vi "Command Editor Dialog _202503.vi"(7 "Name (\"\" to Use Uuid)":string="Event CSM Tiny", 8 "Error In":errorcluster caption="Error in (no error)", 11 "Command":string="UI: Front Panel State >> Open -@ abc") -> (0 "Error Out":errorcluster, 3 "Command Out":string)   [LabVIEW 2017]
uses:
  user.lib/_NEVSTOP/Communicable State Machine(CSM)/AdvanceAPI/CSM - Keywords.vi
  user.lib/_NEVSTOP/Communicable State Machine(CSM)/AdvanceAPI/CSM - Break Down Multiple States String.vi
  user.lib/_NEVSTOP/Communicable State Machine(CSM)/AdvanceAPI/CSM - Compact Multiple States.vi
  user.lib/_NEVSTOP/Communicable State Machine(CSM)/_Polymophic/CSM - Replace Marks in Messages.vi
  user.lib/_NEVSTOP/Communicable State Machine(CSM)/_Polymophic/Add State(s) to Queue By BOOL(Element).vi
  user.lib/_NEVSTOP/Communicable State Machine(CSM)/_Polymophic/Build Message with Arguments(Auto Check).vi
  user.lib/_NEVSTOP/Communicable State Machine(CSM)/Communicable State Machine.lvlib
  user.lib/_NEVSTOP/Communicable State Machine(CSM)/_csmHelper/API with lvcsm Support/CSM-Helper API with lvcsm Support.lvlib
  user.lib/_NEVSTOP/Communicable State Machine(CSM)/_csmHelper/CSM-Helper.lvclass
  user.lib/_NEVSTOP/Communicable State Machine(CSM)/_Shared/CSM Shared.lvlib
panel:
  in  "UserDef State Only":bool
  in  "State":string(combo)
  in  "Argument":string(combo)
  in  "symbol":string(combo)
  in  "Target":string(combo)
  in  "Comments":string
  in  "CSM-VI":string(combo)
  out "current time":timestamp
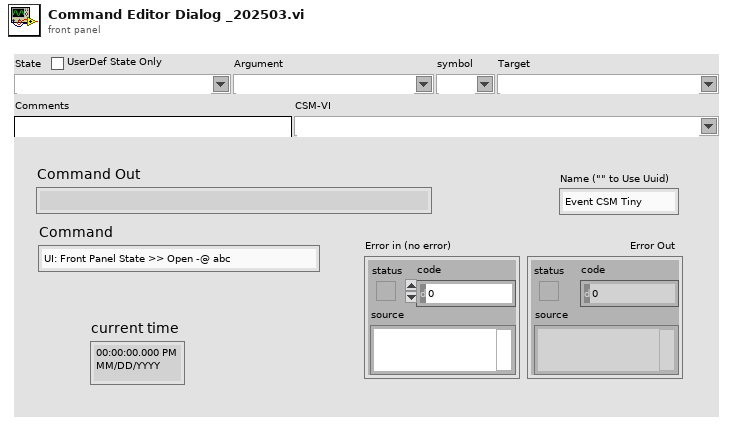
[diagram p1: front panel]
types:
  T1 = enum32{"Invalid", "Standard", "Closed", "Hidden", "Minimized", "Maximized"}
  T2 = enum32{"invalid app kind", "Development System", "Run Time System", "Student Edition", "Embedded LabVIEW", "Evaluation", "Custom"}
  T3 = enum8{"Enabled", "Disabled", "Disabled and Grayed Out"}
  T4 = typedef "Communicable State Machine.lvlib/_CSM_Response Source Message.ctl" = cluster{"‘State":string, "’Arguments":string, "’Error":errorcluster}
  T5 = typedef "eventvkey.ctl" = enum16{"ASCII", "Enter", "Return", "Shift", "Ctrl", "Alt", "Cmd", "Opt", "Caps", "NumLock", "Clear", "Break", "Up", "Down", "Left", "Right", "Insert", "Delete", "Home", "End", "PageUp", "PageDown", "Escape", "Help", "Pause", "ScrollLock", "F1", "F2", "F3", "F4", "F5", "F6", "F7", "F8", "F9", "F10", "F11", "F12", "F13", "F14", "F15", "F16", "F17", "F18", "F19", "F20", "F21", "F22", "F23", "F24", "Play", "VolumeUp", "VolumeDown", "Mute", "Two Byte Char"}
  T6 = cluster{"Shift":bool, "Ctrl":bool, "Alt":bool, "Cmd":bool, "Opt":bool}
  T7 = cluster{"Current VI Reference":refnum<vi>, "Close Panel on Exit?":bool}
  T8 = cluster{"Core":cluster{"Current VI Reference":refnum<vi>, "Close Panel on Exit?":bool}, "Command":string}
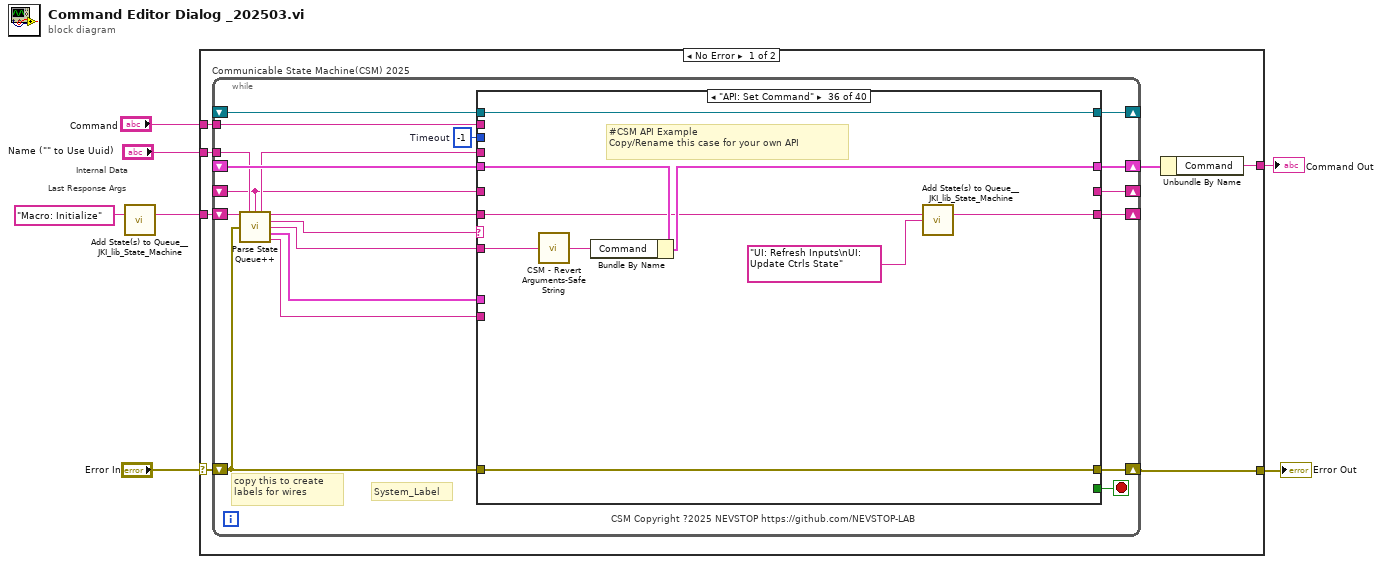
[diagram p0: block diagram]
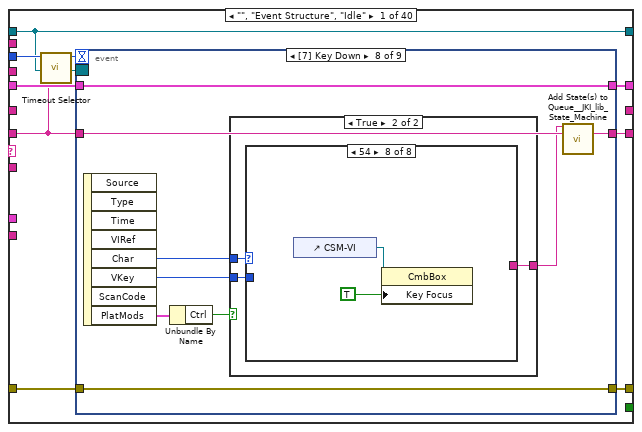
[diagram p2: hidden frame]
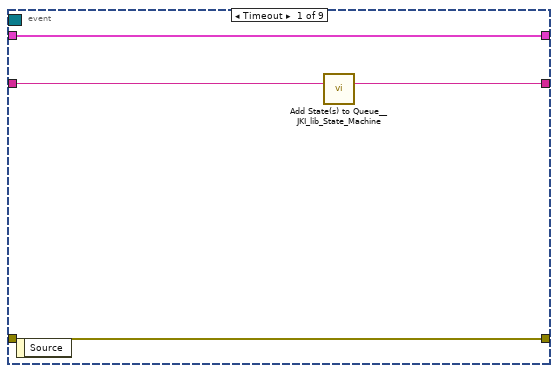
[diagram p3: hidden frame]
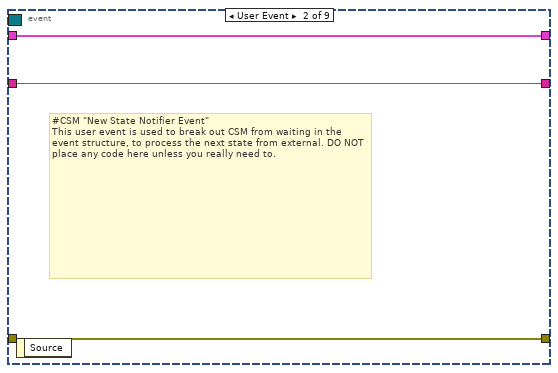
[diagram p4: hidden frame]
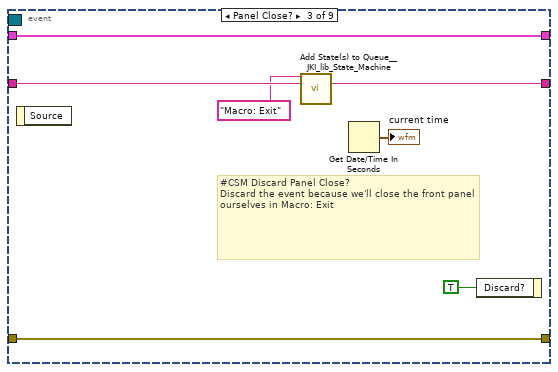
[diagram p5: hidden frame]
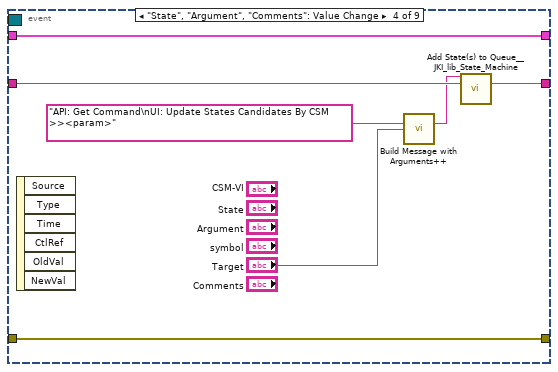
[diagram p6: hidden frame]
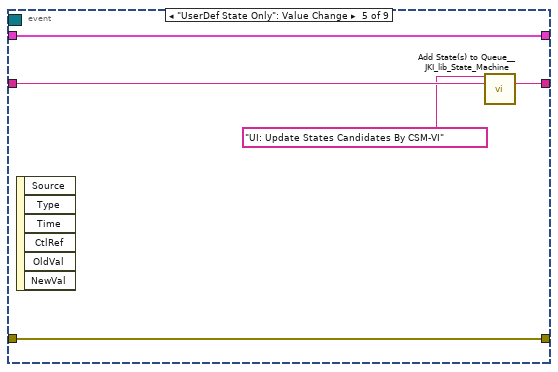
[diagram p7: hidden frame]
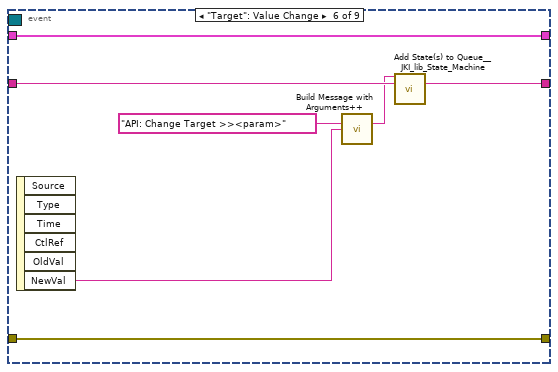
[diagram p8: hidden frame]
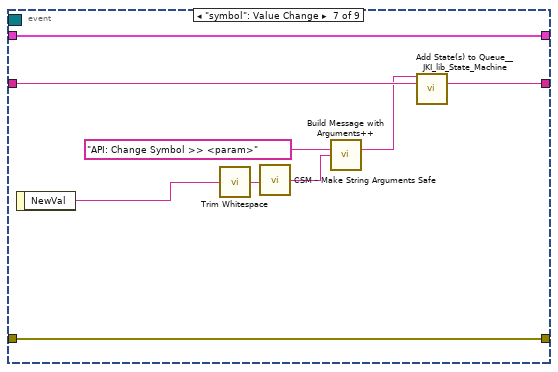
[diagram p9: hidden frame]
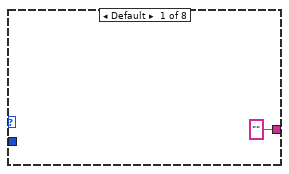
[diagram p11: hidden frame]
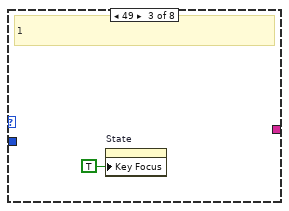
[diagram p13: hidden frame]
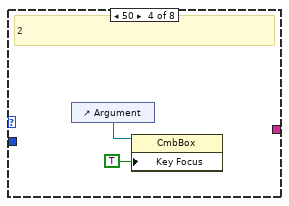
[diagram p14: hidden frame]
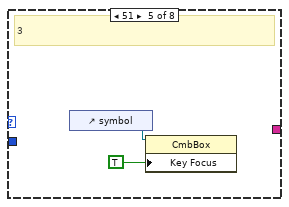
[diagram p15: hidden frame]
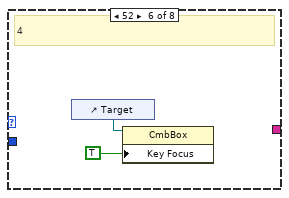
[diagram p16: hidden frame]
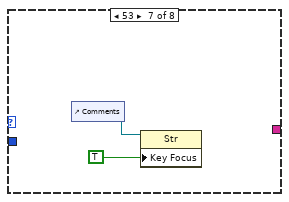
[diagram p17: hidden frame]
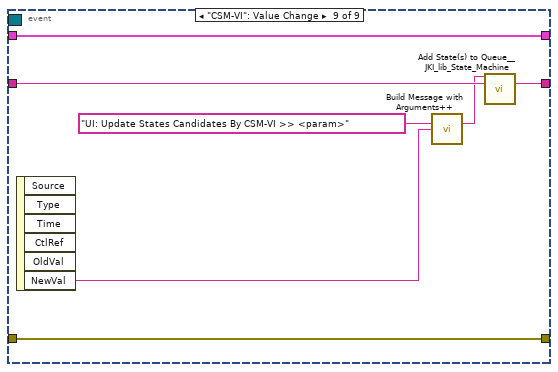
[diagram p18: hidden frame]
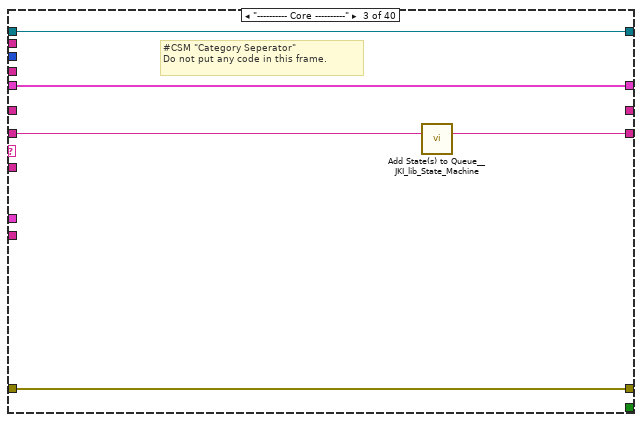
[diagram p20: hidden frame]
diagram:
  # "Last Response Args"
  # "Internal Data"
  n1 = call <vilib>:"Add State(s) to Queue__JKI_lib_State_Machine.vi"("State(s) in (\"\")"="Macro: Initialize" ("Init State(\"Macro: Initialize\")")) -> ("States Out"=w7:string)  [unwired: 14 in]
  n2 = case shown="No Error" "Error In" {
    selector: "Error In" -> [w11 w534]
    tunnel: w7 -> [w14 _]
    tunnel: "Name (\"\" to Use Uuid)" -> [w13 _]
    tunnel: [w12 w534] -> w4
    tunnel: [w9 w533] -> w1
    tunnel: "Command" -> [w8 w533]
    frame No Error {
      n3 = while "Communicable State Machine(CSM) 2025" {
        shift-right: [w29] -> w10
        shift-left: _ -> [w28]
        shift-right: [w32] -> w12
        shift-left: w11 -> [w26]
        shift-right: [w31] -> _
        shift-left: w14 -> [w33]
        tunnel: w13 -> [w22]
        shift-right: [w25] -> _
        shift-left: _ -> [w16]
        shift-right: [w24] -> _
        shift-left: _ -> [w23]
        tunnel: w8 -> [w15]
        stop <- w30 stop-if-true
        w27 = -1  # Timeout
        # "copy this to create labels for wires"
        # "System_Label"
        # "CSM Copyright ?2025 NEVSTOP https://github.com/NEVSTOP-LAB"
        n4 = call "Parse State Queue++.vi"("State Queue"=w33, "Name (\"\" to Use UUID)"=w22, "Response Arguments"=w16, "Previous Error"=w26) -> ("Name Used"=w17:string, "Remaining States"=w34:string, "Current State"=w21:string, "Arguments"=w20:string, "Additional Information"=w19:T4, "Source CSM"=w18:string)  [unwired: 6 in]
        n5 = case shown="\"API: Set Command\"" w21 {
          selector: w21 -> [_ _ _ w128 _ _ _ _ _ _ _ _ _ _ _ _ _ _ _ _ _ _ _ _ _ _ _ _ _ _ _ _ _ _ _ _ _ _ _ _]
          tunnel: w34 -> [w35 w119 w125 w133 w140 w146 w169 w175 w182 w191 w204 w219 w225 w230 w237 w244 w249 w256 w260 w266 w272 w278 w298 w314 w383 w388 w395 w413 w422 w429 w445 w456 w462 w474 w477 w480 w501 w513 w523 w532]
          tunnel: w20 -> [_ _ _ _ _ w145 w164 w174 w181 w190 _ _ _ _ _ _ _ _ _ _ _ _ w293 w308 _ _ w397 w410 w419 w426 _ _ _ _ _ w482 _ w514 w520 _]
          tunnel: w28 -> [w42 w118 w122 w131 w139 w150 w170 w177 w184 w193 w203 w212 w223 w227 _ w239 w246 w255 w259 w263 w268 w281 w296 w310 w382 w387 w399 w412 w421 w428 w444 w453 w459 w471 w476 w486 w500 w516 w525 w529]
          tunnel: [w41 w120 w123 w126 w141 errorcluster {"status"=FALSE, "code"=0, "source"=""} ("error out") w165 w172 w179 w196 w205 w216 w222 w228 w234 w240 w247 w250 w258 w264 w270 w291 w294 w311 w384 w389 w400 w414 w423 w430 w446 w454 w460 w472 w478 w487 w502 w517 w526 w530] -> w32
          tunnel: w26 -> [w40 w120 w123 w134 w141 w147 w171 w173 w180 _ w205 w216 w222 w228 w234 w241 w247 _ w261 w264 w270 w291 w295 w312 w384 w389 w400 w414 w423 w430 w446 w454 w460 w472 w478 w487 w502 w517 w526 w530]
          tunnel: [w43 w119 w124 w132 w140 w142 w168 w178 w185 w192 w204 w218 w224 w229 w236 w243 w248 w256 w260 w265 w271 w279 w297 w313 w383 w388 w396 w413 w422 w429 w445 w455 w461 w473 w477 w481 w501 w512 w527 w531] -> w31
          tunnel: [_ _ _ _ _ _ TRUE _ _ _ _ _ TRUE _ _ _ _ _ _ _ _ _ _ _ _ _ _ _ _ _ _ _ _ _ _ _ _ _ _ _] -> w30
          tunnel: [w39 w118 w122 w131 w139 w150 w170 w177 w184 w194 w203 w217 w223 w227 w235 w239 w246 w255 w259 w263 w268 w281 w296 w310 w382 w387 w399 w412 w421 w428 w444 w453 w459 w471 w476 w484 w490 w516 w525 w529] -> w29
          tunnel: w27 -> [w38 _ _ _ _ _ _ _ _ _ _ _ _ _ _ _ _ _ _ _ _ _ _ _ _ _ _ _ _ _ _ _ _ _ _ _ _ _ _ _]
          tunnel: w18 -> [_ _ _ _ _ _ _ _ _ w188 _ _ _ _ _ _ _ _ _ _ _ _ _ _ _ _ _ _ _ _ _ _ _ _ _ _ _ _ _ _]
          tunnel: w19 -> [_ _ _ _ _ _ _ _ _ w195 _ _ _ _ _ _ _ _ _ _ _ _ _ _ _ _ _ _ _ _ _ _ _ _ _ _ _ _ _ _]
          tunnel: [_ _ _ "" w135 _ _ _ _ _ _ _ _ _ _ _ _ _ _ _ _ _ _ _ _ _ _ _ _ _ _ _ _ _ _ _ w495 _ _ _] -> w25
          tunnel: [w37 w117 w121 w129 w138 w149 w166 w176 w183 w197 w202 w206 w220 w226 w232 w238 w245 w254 w257 w262 w269 w290 w292 w307 w381 w386 w398 w411 w420 w427 w443 w452 w457 w464 w475 w485 w499 w515 w524 w528] -> w24
          tunnel: w23 -> [w37 w117 w121 w129 w138 w149 w166 w176 w183 w197 w202 w206 w220 w226 w232 w238 w245 _ w257 w262 w269 w290 w292 w307 w381 w386 w398 w411 w420 w427 w443 w452 w457 w464 w475 w485 w499 w515 w524 w528]
          tunnel: w17 -> [_ _ _ w127 _ _ w163 _ _ _ _ _ _ _ _ _ _ w253 _ _ _ _ _ _ _ _ _ _ _ _ _ _ _ _ _ _ _ _ _ _]
          tunnel: w16 -> [_ _ _ _ _ _ _ _ _ _ _ _ _ _ _ _ _ _ _ _ _ _ _ _ _ _ _ _ _ _ _ _ _ _ _ _ _ _ _ _]
          tunnel: w15 -> [_ _ _ _ _ _ _ _ _ _ _ _ _ _ w231 _ _ _ _ _ _ _ _ _ _ _ _ _ _ _ _ _ _ _ _ _ _ _ _ _]
          frame "", "Event Structure", "Idle" {
            n6 = call "Timeout Selector.vi"("Remaining States"=w35, "Timeout Expected"=w38) -> ("Timeout"=w36:i32)  [unwired: 5 in]
            n7 = event shown="[7] Key Down" {
              selector: w37 -> [_ _ _ _ _ _ _ _ _]
              dyn-events: _ -> [_ _ _ _ _ _ _ _ _]
              timeout: w36 -> [_ _ _ _ _ _ _ _ _]
              tunnel: w35 -> [w47 w49 w57 w61 w66 w73 w82 w88 w113]
              tunnel: [w46 w49 w56 w62 w67 w74 w83 w89 w114] -> w43
              tunnel: w42 -> [w44 w50 w54 w63 w68 w75 w84 w93 w115]
              tunnel: [w45 w48 w55 w64 w69 w76 w85 w94 w116] -> w41
              tunnel: w40 -> [w45 w48 w55 w64 w69 w76 w85 w94 w116]
              tunnel: [w44 w50 w54 w63 w68 w75 w84 w93 w115] -> w39
              event Timeout {
                n8 = event-data() -> ()  [unwired: 1 in, 1 out]
                n9 = call <vilib>:"Add State(s) to Queue__JKI_lib_State_Machine.vi"("State(s) in (\"\")"=w47) -> ("States Out"=w46:string)  [unwired: 14 in]
              }
              event User Event {
                # "#CSM \"New State Notifier Event\"\nThis user event is used to break out CSM from waiting in the event structure, to process the next state from external. DO NOT place any code here unless you really need to."
                n10 = event-data() -> ()  [unwired: 1 in, 1 out]
              }
              event Panel Close? {
                # "#CSM Discard Panel Close?\nDiscard the event because we'll close the front panel ourselves in Macro: Exit"
                n11 = event-data() -> ()  [unwired: 1 in, 1 out]
                n12 = call <vilib>:"Add State(s) to Queue__JKI_lib_State_Machine.vi"("State(s) in Front (\"\")"="Macro: Exit", "State(s) in (\"\")"=w57) -> ("States Out"=w56:string)  [unwired: 13 in]
                n13 = Get Date/Time In Seconds() -> (seconds since 1Jan1904=→"current time":timestamp)
                n14 = event-data("Discard?"=TRUE) -> ()  [unwired: 1 in, 1 out]
              }
              event "State", "Argument", "Comments": Value Change {
                n15 = event-data() -> ()  [unwired: 1 in, 6 out]
                n16 = call-poly "Build Message with Arguments++.vi"("States With Replace Token"="API: Get Command\nUI: Update States Candidates By CSM >><param>" ("State(s) in Front (\"\")"), "<param>"="Target") -> ("States"=w59:string)  [unwired: 13 in]
                n17 = call <vilib>:"Add State(s) to Queue__JKI_lib_State_Machine.vi"("State(s) in Front (\"\")"=w59, "State(s) in (\"\")"=w61) -> ("States Out"=w62:string)  [unwired: 13 in]
              }
              event "UserDef State Only": Value Change {
                n18 = event-data() -> ()  [unwired: 1 in, 6 out]
                n19 = call <vilib>:"Add State(s) to Queue__JKI_lib_State_Machine.vi"("State(s) in Front (\"\")"="UI: Update States Candidates By CSM-VI" ("State(s) in Front (\"\")"), "State(s) in (\"\")"=w66) -> ("States Out"=w67:string)  [unwired: 13 in]
              }
              event "Target": Value Change {
                n20 = event-data() -> ("NewVal"=w70:string)  [unwired: 1 in, 5 out]
                n21 = call-poly "Build Message with Arguments++.vi"("States With Replace Token"="API: Change Target >><param>" ("State(s) in Front (\"\")"), "<param>"=w70) -> ("States"=w71:string)  [unwired: 13 in]
                n22 = call <vilib>:"Add State(s) to Queue__JKI_lib_State_Machine.vi"("State(s) in Front (\"\")"=w71, "State(s) in (\"\")"=w73) -> ("States Out"=w74:string)  [unwired: 13 in]
              }
              event "symbol": Value Change {
                n23 = event-data() -> ("NewVal"=w77:string)  [unwired: 1 in]
                n24 = call <vilib>:"Trim Whitespace.vi"("string"=w77) -> ("trimmed string"=w78:string)  [unwired: 1 in]
                n25 = call "CSM - Make String Arguments Safe.vi"("Argument String"=w78) -> ("Safe Argument String"=w79:string)  [unwired: 8 in]
                n26 = call-poly "Build Message with Arguments++.vi"("States With Replace Token"="API: Change Symbol >> <param>" ("State(s) in Front (\"\")"), "<param>"=w79) -> ("States"=w80:string)  [unwired: 13 in]
                n27 = call <vilib>:"Add State(s) to Queue__JKI_lib_State_Machine.vi"("State(s) in Front (\"\")"=w80, "State(s) in (\"\")"=w82) -> ("States Out"=w83:string)  [unwired: 13 in]
              }
              event Key Down {
                n28 = event-data() -> ("Char"=w91:i16, "VKey"=w86:T5, "PlatMods"=w92:T6)  [unwired: 1 in, 5 out]
                n29 = Unbundle By Name(w92) -> ("Ctrl"=w90:bool)
                n30 = case shown="True" w90 {
                  tunnel: w91 -> [_ w97]
                  tunnel: [_ w96] -> w87
                  tunnel: w86 -> [_ w95]
                  frame False {
                  }
                  frame True {
                    n31 = case shown="54" w97 {
                      tunnel: ["" ("State with Arguments") _ _ _ _ _ _ _] -> w96
                      tunnel: w95 -> [_ _ _ _ _ _ _ _]
                      frame Default {
                      }
                      frame 0 {
                      }
                      frame 49 {
                        # "1"
                        n32 = property on="State" class="CmbBox"("Key Focus"=TRUE) -> ()  [unwired: 2 in, 2 out]
                      }
                      frame 50 {
                        # "2"
                        n33 = control-ref of="Argument"() -> (w101:refnum<vi>)
                        n34 = property on="Property Node" class="CmbBox"(reference=w101, "Key Focus"=TRUE) -> ()  [unwired: 1 in, 2 out]
                      }
                      frame 51 {
                        # "3"
                        n35 = control-ref of="symbol"() -> (w103:refnum<vi>)
                        n36 = property on="Property Node" class="CmbBox"(reference=w103, "Key Focus"=TRUE) -> ()  [unwired: 1 in, 2 out]
                      }
                      frame 52 {
                        # "4"
                        n37 = control-ref of="Target"() -> (w105:refnum<vi>)
                        n38 = property on="Property Node" class="CmbBox"(reference=w105, "Key Focus"=TRUE) -> ()  [unwired: 1 in, 2 out]
                      }
                      frame 53 {
                        n39 = control-ref of="Comments"() -> (w107:refnum<vi>)
                        n40 = property on="Property Node" class="Str"(reference=w107, "Key Focus"=TRUE) -> ()  [unwired: 1 in, 2 out]
                      }
                      frame 54 {
                        n41 = control-ref of="CSM-VI"() -> (w109:refnum<vi>)
                        n42 = property on="Property Node" class="CmbBox"(reference=w109, "Key Focus"=TRUE) -> ()  [unwired: 1 in, 2 out]
                      }
                    }
                  }
                }
                n43 = call <vilib>:"Add State(s) to Queue__JKI_lib_State_Machine.vi"("State(s) in Front (\"\")"=w87, "State(s) in (\"\")"=w88) -> ("States Out"=w89:string)  [unwired: 13 in]
              }
              event "CSM-VI": Value Change {
                n44 = event-data() -> ("NewVal"=w110:string)  [unwired: 1 in, 5 out]
                n45 = call-poly "Build Message with Arguments++.vi"("States With Replace Token"="UI: Update States Candidates By CSM-VI >> <param>" ("State(s) in Front (\"\")"), "<param>"=w110) -> ("States"=w111:string)  [unwired: 13 in]
                n46 = call <vilib>:"Add State(s) to Queue__JKI_lib_State_Machine.vi"("State(s) in Front (\"\")"=w111, "State(s) in (\"\")"=w113) -> ("States Out"=w114:string)  [unwired: 13 in]
              }
            }
          }
          frame "CSM Documentation" {
            # "#CSM README FIRST\n\nCommunicable State Machine(CSM) is a LabVIEW application framework that builds upon JKI State Machine(JKISM). It follows the pattern of JKISM and extends the keywords to describe message communication between modules, including concepts such as Sync-Message, Async-Message, Subscription/Unsubscription of status - essential elements for creating reusable code modules. For more information, please visit the CSM wiki: https://nevstop-lab.github.io/CSM-Wiki/\n\nFor instructions on JKI State Machine, visit: http://jki.net/state-machine/\nFor information about CSM, visit: https://github.com/NEVSTOP-LAB"
            # "#CSM \"Documentation\"\nCase for holding CSM Documenation"
          }
          frame "---------- Core ----------" {
            # "#CSM \"Category Seperator\"\nDo not put any code in this frame."
            n47 = call <vilib>:"Add State(s) to Queue__JKI_lib_State_Machine.vi"("State(s) in (\"\")"=w125) -> ("States Out"=w124:string)  [unwired: 14 in]
          }
          frame Default {
            # "#CSM \"Default\"\nthis is used to capture unhandled states and typos"
            # "Handle mistyped state name (developer tool)"
            n48 = call "CSM Unhandled State Error.vi"("error in (no error)"=w134, "Undefined State"=w128, "CSM Name"=w127) -> ("error out"=w126:errorcluster)  [unwired: 8 in]
            n49 = call <vilib>:"Add State(s) to Queue__JKI_lib_State_Machine.vi"("State(s) in (\"\")"=w133) -> ("States Out"=w132:string)  [unwired: 14 in]
          }
          frame "VI Reference" {
            n50 = Unbundle By Name(w139) -> ("Core"=w137:T7)
            n51 = Unbundle By Name(w137) -> ("Current VI Reference"=w136:refnum<vi>)
            n52 = call "CSM - Convert Data to HexStr.vi"("Variant"=w136) -> ("HEX String (0-9,A-F)"=w135:string)  [unwired: 8 in]
          }
          frame "Error Handler" {
            # "#CSM Disable this error dialog if you need"
            # "#CSM \"Error Handler\"\nYou can also output any states to clean-up after errors occur"
            # "Clear error"
            n53 = case shown="Error" w147 {
              selector: w147 -> [_ w157]
              tunnel: [w156 w159] -> w143
              tunnel: w146 -> [w156 w158]
              tunnel: w145 -> [w155 _]
              tunnel: [w154 w157] -> w148
              frame No Error {
                n54 = call "CSM - Convert Argument to Error.vi"("Argument"=w155) -> ("Error"=w154:errorcluster)  [unwired: 4 in]
                n55 = flat-sequence {
                  frame #0 {
                    # "#CSM External Error Handler Case\nUsually, it's because This CSM register others' \"Error Occurred\" status with \"Error Handler\". If other CSM have any error, the error will be passed here for central handling."
                  }
                }
              }
              frame Error {
                # "#CSM Internal Error Handler Case \nIf any error Occurred, \"Error Occurred\" \nstatus update will be broadcasted to system.\nParameter is Error Cluster."
                n56 = call "CSM - Convert Error to Argument.vi"("Error"=w157) -> ("Argument"=w161:string)  [unwired: 4 in]
                n57 = call <vilib>:"Build State String with Arguments__JKI_lib_State_Machine.vi"("Arguments (\"\")"=w161, "State"="Error Occurred" ("Status with Arguments")) -> ("State with Arguments"=w160:string)  [unwired: 4 in]
                n58 = call "CSM - Broadcast Status Change.vi"("Status With Arguments"=w160, "State Queue"=w158) -> ("Remaining States"=w159:string)  [unwired: 13 in]
              }
            }
            n59 = disable-structure shown="Enabled" {
              disable-tunnel: w148 -> [w152 w153]
              frame Enabled {
                n60 = call <vilib>:"General Error Handler.vi"("error in (no error)"=w152) -> ()  [unwired: 10 in, 5 out]
              }
              frame Disabled {
                n61 = call <vilib>:"Clear Errors.vi"("error in (no error)"=w153) -> ()  [unwired: 5 in, 2 out]
              }
            }
            n62 = call <vilib>:"Add State(s) to Queue__JKI_lib_State_Machine.vi"("State(s) in Front (\"\")"="// Post Error States", "State(s) in (\"\")"=w143) -> ("States Out"=w142:string)  [unwired: 13 in]
          }
          frame "Critical Error" {
            # "#CSM Stop in Critical Error\nWhen Critical Error occurs, Stop the loop immediately. Do NOT change this unless you fully understand the impact."
            # "#CSM \"Critical Error\"\nWhen any un-recoverable error occurs, CSM goes into this case."
            n63 = call "CSM Critical Error.vi"("error in (no error)"=w171, "Arugments (As Reason)"=w164, "CSM Name"=w163) -> ("error out"=w165:errorcluster)  [unwired: 8 in]
            n64 = call <vilib>:"Add State(s) to Queue__JKI_lib_State_Machine.vi"("State(s) in (\"\")"=w169) -> ("States Out"=w168:string)  [unwired: 14 in]
          }
          frame "Target Error" {
            # "#CSM \"Target Error\"\nWhen This CSM try to communicate with an un-existed CSM, This CSM goes into this case."
            n65 = call "CSM Target Error.vi"("error in (no error)"=w173, "Arguments (As CSM Name)"=w174) -> ("error out"=w172:errorcluster)  [unwired: 9 in]
            n66 = call <vilib>:"Add State(s) to Queue__JKI_lib_State_Machine.vi"("State(s) in (\"\")"=w175) -> ("States Out"=w178:string)  [unwired: 14 in]
          }
          frame "Target Timeout Error" {
            # "#CSM \"Target Timeout Error\"\nWhen This CSM could not get the sync-call response in time, This CSM goes into this case."
            n67 = call "CSM Target Timeout Error.vi"("error in (no error)"=w180, "Arguments (As CSM Name)"=w181) -> ("error out"=w179:errorcluster)  [unwired: 9 in]
            n68 = call <vilib>:"Add State(s) to Queue__JKI_lib_State_Machine.vi"("State(s) in (\"\")"=w182) -> ("States Out"=w185:string)  [unwired: 14 in]
          }
          frame "Async Response", "Response" {
            n69 = Unbundle(w195) -> ("‘State"=w189:string, "’Arguments"=w187:string, "’Error"=w186:errorcluster)
            n70 = case shown="Default" w189 {
              tunnel: [w201] -> w196
              tunnel: w186 -> [w201]
              tunnel: [w200] -> w194
              tunnel: w193 -> [w200]
              tunnel: [w198] -> w192
              tunnel: w191 -> [w199]
              tunnel: w190 -> [_]
              tunnel: w188 -> [_]
              tunnel: w187 -> [_]
              frame Default {
                # "#CSM Response Comments\nAfter Message is executed, CSM goes to this state for receive the response.\n    For Async Message(->), \"Async Response\" is used. This CSM will goes to \"Async Message Posted\" immediately and receive the \"Async Response\" after the callee finishes the message.\n    For Sync Message(@),  This CSM will wait until the message is done and immediately goes to \"Response\""
                # "#CSM \"Async Response\"\nHandle Async-call Response (\"Async Response\" for ->)"
                # "#CSM \"Response\"\nHandle Sync-call Response (\"Response\" for -@)"
                n71 = call <vilib>:"Add State(s) to Queue__JKI_lib_State_Machine.vi"("State(s) in (\"\")"=w199) -> ("States Out"=w198:string)  [unwired: 14 in]
              }
            }
          }
          frame "Async Message Posted" {
            # "#CSM \"Async Message Posted\"\nAfter Async Message is posted (-> or ->| ), CSM goes to this state for post-action.\nYou can use Argument - State to tell which Async Message is called."
          }
          frame "Initialize Core Data" {
            # "#CSM \"Initialize Core Data\"\nThis is used to determine panel behavior on exit"
            # "originally closed?"
            # "exe?"
            # "If panel starts closed or is an EXE, then close it when we exit"
            n72 = property class="VI"() -> ("FP.State"=w209:T1)  [unwired: 2 in, 2 out]
            n73 = property class="App"() -> ("App.Kind"=w215:T2)  [unwired: 2 in, 2 out]
            n74 = control-ref of="Current VI Reference"() -> (w210:refnum<vi>)
            n75 = Equal?(x=w209, y=T1."Closed" ("Front Panel Window:State")) -> (x = y?=w207:bool)
            n76 = Equal?(x=w215, y=T2."Run Time System" ("Application:Kind")) -> (x = y?=w213:bool)
            n77 = Or(x=w207, y=w213) -> (x .or. y?=w211:bool)
            n78 = Bundle By Name(cluster=w212, "Core.Current VI Reference"=w210, "Core.Close Panel on Exit?"=w211) -> (w217:T8)
            n79 = call <vilib>:"Add State(s) to Queue__JKI_lib_State_Machine.vi"("State(s) in (\"\")"=w219) -> ("States Out"=w218:string)  [unwired: 14 in]
          }
          frame "Exit" {
            # "#CSM \"Exit\"\nCase for exiting the loop. No errors that occur here will be handled."
            n80 = call <vilib>:"Add State(s) to Queue__JKI_lib_State_Machine.vi"("State(s) in (\"\")"=w225) -> ("States Out"=w224:string)  [unwired: 14 in]
          }
          frame "---------- Data ----------" {
            # "#CSM \"Category Seperator\"\nDo not put any code in this frame."
            n81 = call <vilib>:"Add State(s) to Queue__JKI_lib_State_Machine.vi"("State(s) in (\"\")"=w230) -> ("States Out"=w229:string)  [unwired: 14 in]
          }
          frame "Data: Initialize" {
            w233 = T7 {"Current VI Reference"=refnum, "Close Panel on Exit?"=FALSE}  # Core
            n82 = Bundle("Core"=w233, "Command"=w231) -> (w235:T8)  [unwired: 1 in]
            n83 = call <vilib>:"Add State(s) to Queue__JKI_lib_State_Machine.vi"("State(s) in (\"\")"=w237) -> ("States Out"=w236:string)  [unwired: 14 in]
          }
          frame "Data: Cleanup" {
            # "Cleanup any data and references, here.\n(this is called automatically, by the Macro: Exit)"
            n84 = Unbundle By Name(w239) -> ("Core.Current VI Reference"=w242:refnum<vi>)
            n85 = Close Reference(reference=w242, error in (no error)=w241) -> (error out=w240:errorcluster)
            n86 = call <vilib>:"Add State(s) to Queue__JKI_lib_State_Machine.vi"("State(s) in (\"\")"=w244) -> ("States Out"=w243:string)  [unwired: 14 in]
          }
          frame "---------- Events ----------" {
            # "#CSM \"Category Seperator\"\nDo not put any code in this frame."
            n87 = call <vilib>:"Add State(s) to Queue__JKI_lib_State_Machine.vi"("State(s) in (\"\")"=w249) -> ("States Out"=w248:string)  [unwired: 14 in]
          }
          frame "Events: Register" {
            # "#CSM \"Events: Register\"\nRegister user event. New Message Event is registered to break CSM waiting in event structure by default."
            # "#CSM Register New Message Event\nRegister message event to break Waiting in Event structure."
            n88 = call "CSM - Get New State Notifier Event.vi"("Name (\"\" to Use UUID)"=w253) -> ("error out"=w251:errorcluster, "New State Notifier Event"=w252:refnum<user-event>)  [unwired: 9 in]
            n89 = register-events(error in=w251, w252) -> (reference out=w254:refnum<event-registration>, error out=w250:errorcluster)  [unwired: 1 in]
          }
          frame "Events: Unregister" {
            # "#CSM \"Events: Unregister\"\nUnregister user event."
            n90 = Unregister For Events(event registration refnum=w257, error in=w261) -> (error out=w258:errorcluster)
          }
          frame "---------- UI ----------" {
            # "#CSM \"Category Seperator\"\nDo not put any code in this frame."
            n91 = call <vilib>:"Add State(s) to Queue__JKI_lib_State_Machine.vi"("State(s) in (\"\")"=w266) -> ("States Out"=w265:string)  [unwired: 14 in]
          }
          frame "UI: Initialize" {
            # "#CSM \"UI: Initialize\"\nInitialize the User Interface, here.\n(this is called automatically, by the Macro: Init)"
            n92 = local write "UserDef State Only"(TRUE ("UserDef State Only")) -> ()
            n93 = call <vilib>:"Add State(s) to Queue__JKI_lib_State_Machine.vi"("State(s) in (\"\")"=w272) -> ("States Out"=w271:string)  [unwired: 14 in]
          }
          frame "UI: Refresh Inputs" {
            n94 = Unbundle By Name(w281) -> ("Command"=w280:string)
            n95 = call "Remove Comments from Single-line.vi"("single-line text"=w280) -> ("single-line text without comments"=w286:string)  [unwired: 2 in]
            n96 = call "Split Single-line Message.vi"("single-line text"=w286) -> ("operator"=w275:string, "state"=w289:string, "args"=w288:string, "source/target"=w274:string)  [unwired: 6 in]
            n97 = String Length(string=w286) -> (length=w287:i32)
            n98 = String Subset(string=w280, offset (0)=w287) -> (substring=w284:string)  [unwired: 1 in]
            n99 = call "Trim Single-line Text.vi"("single-line text"=w284) -> ("trimed text"=w283:string)  [unwired: 2 in]
            n100 = call "CSM - Make String Arguments Safe.vi"("Argument String"=w275) -> ("Safe Argument String"=w273:string)  [unwired: 8 in]
            n101 = Match Pattern(string=w283, regular expression="^[/][/]+") -> (after substring=w285:string)  [unwired: 1 in, 3 out]
            n102 = call-poly "Build Message with Arguments++.vi"("States With Replace Token"="API: Change Target >> <1>\nAPI: Change Symbol >> <2>\nUI: Update Ctrls State" ("State(s) in Front (\"\")"), "<1>"=w274, "<2>"=w273) -> ("States"=w276:string)  [unwired: 12 in]
            n103 = local write "Comments"(w285) -> ()
            n104 = local write "State"(w289) -> ()
            n105 = local write "Argument"(w288) -> ()
            n106 = local write "Target"(w274) -> ()
            n107 = call <vilib>:"Add State(s) to Queue__JKI_lib_State_Machine.vi"("State(s) in Front (\"\")"=w276, "State(s) in (\"\")"=w278) -> ("States Out"=w279:string)  [unwired: 13 in]
          }
          frame "UI: Cursor Set" {
            # "#CSM \"UI: Cursor Set\"\nSet and Unset Cursor Busy.\n(Usage: \"UI: Cursor Set >> Busy|Idle\")"
            # "Argument"
            n108 = disable-structure shown="Default" {
              disable-tunnel: w295 -> [w301 w306]
              disable-tunnel: [w300 w306] -> w294
              disable-tunnel: w293 -> [w299 _]
              frame condition #0 (active) {
                n109 = case shown="\"Idle\", Default" w299 {
                  tunnel: w301 -> [w303 w305]
                  tunnel: [w302 w304] -> w300
                  frame "Idle", Default {
                    n110 = call <vilib>:"Unset Busy.vi"("error in (no error)"=w303) -> ("error out"=w302:errorcluster)  [unwired: 10 in]
                  }
                  frame "Busy" {
                    n111 = call <vilib>:"Set Busy.vi"("error in (no error)"=w305) -> ("error out"=w304:errorcluster)  [unwired: 9 in, 1 out]
                  }
                }
              }
              frame condition #1 {
              }
            }
            n112 = call <vilib>:"Add State(s) to Queue__JKI_lib_State_Machine.vi"("State(s) in (\"\")"=w298) -> ("States Out"=w297:string)  [unwired: 14 in]
          }
          frame "UI: Front Panel State" {
            # "#CSM \"UI: Front Panel State\"\nSet Front Panel Open or Closed\n(Usage: \"UI: Front Panel State >> Open|Close\")"
            # "Argument"
            n113 = Unbundle By Name(w310) -> ("Core.Current VI Reference"=w309:refnum<vi>)
            n114 = call <vilib>:"Add State(s) to Queue__JKI_lib_State_Machine.vi"("State(s) in (\"\")"=w314) -> ("States Out"=w313:string)  [unwired: 14 in]
            n115 = case shown="\"Close\", \"Closed\"" w308 {
              tunnel: w312 -> [w320 w335 w346 w359 w372]
              tunnel: [w322 w336 w348 w361 w374] -> w311
              tunnel: w309 -> [w321 w333 w347 w360 w373]
              frame "Open", "Standard", Default {
                w315 = T1."Standard" ("State")
                n116 = property class="VI"(reference=w321, error in=w320) -> (reference out=w318:refnum<vi>, error out=w319:errorcluster, "FP.State"=w317:T1)
                n117 = Not Equal?(x=w317, y=w315) -> (x != y?=w316:bool)
                n118 = case shown="True" w316 {
                  tunnel: [w326 w328] -> w322
                  tunnel: w319 -> [w325 w328]
                  tunnel: w318 -> [w324 _]
                  tunnel: w315 -> [w323 _]
                  frame True {
                    n119 = invoke class="VI" method="FP.Open"(reference=w324, error in=w325, "Activate"=TRUE, "State"=w323) -> (error out=w326:errorcluster)  [unwired: 1 in, 4 out]
                  }
                  frame False {
                  }
                }
              }
              frame "Close", "Closed" {
                n120 = property class="VI"(reference=w333, error in=w335) -> (reference out=w332:refnum<vi>, error out=w334:errorcluster, "FP.State"=w330:T1)
                n121 = Not Equal?(x=w330, y=T1."Closed" ("Front Panel Window:State")) -> (x != y?=w329:bool)
                n122 = case shown="False" w329 {
                  tunnel: [w337 w340] -> w336
                  tunnel: w334 -> [w337 w339]
                  tunnel: w332 -> [_ w338]
                  frame False {
                  }
                  frame True {
                    n123 = invoke class="VI" method="FP.Close"(reference=w338, error in=w339) -> (error out=w340:errorcluster)  [unwired: 1 in, 2 out]
                  }
                }
              }
              frame "Hidden", "Hide" {
                w341 = T1."Hidden" ("State")
                n124 = property class="VI"(reference=w347, error in=w346) -> (reference out=w344:refnum<vi>, error out=w345:errorcluster, "FP.State"=w343:T1)
                n125 = Not Equal?(x=w343, y=w341) -> (x != y?=w342:bool)
                n126 = case shown="True" w342 {
                  tunnel: [w352 w353] -> w348
                  tunnel: w345 -> [w351 w353]
                  tunnel: w344 -> [w350 _]
                  tunnel: w341 -> [w349 _]
                  frame True {
                    n127 = invoke class="VI" method="FP.Open"(reference=w350, error in=w351, "State"=w349) -> (error out=w352:errorcluster)  [unwired: 2 in, 4 out]
                  }
                  frame False {
                  }
                }
              }
              frame "Minimize", "Minimized" {
                w354 = T1."Minimized" ("State")
                n128 = property class="VI"(reference=w360, error in=w359) -> (reference out=w357:refnum<vi>, error out=w358:errorcluster, "FP.State"=w356:T1)
                n129 = Not Equal?(x=w356, y=w354) -> (x != y?=w355:bool)
                n130 = case shown="True" w355 {
                  tunnel: [w365 w366] -> w361
                  tunnel: w358 -> [w364 w366]
                  tunnel: w357 -> [w363 _]
                  tunnel: w354 -> [w362 _]
                  frame True {
                    n131 = invoke class="VI" method="FP.Open"(reference=w363, error in=w364, "State"=w362) -> (error out=w365:errorcluster)  [unwired: 2 in, 4 out]
                  }
                  frame False {
                  }
                }
              }
              frame "Maximize", "Maximized" {
                w367 = T1."Maximized" ("State")
                n132 = property class="VI"(reference=w373, error in=w372) -> (reference out=w370:refnum<vi>, error out=w371:errorcluster, "FP.State"=w369:T1)
                n133 = Not Equal?(x=w369, y=w367) -> (x != y?=w368:bool)
                n134 = case shown="True" w368 {
                  tunnel: [w378 w379] -> w374
                  tunnel: w371 -> [w377 w379]
                  tunnel: w370 -> [w376 _]
                  tunnel: w367 -> [w375 _]
                  frame True {
                    n135 = invoke class="VI" method="FP.Open"(reference=w376, error in=w377, "State"=w375) -> (error out=w378:errorcluster)  [unwired: 2 in, 4 out]
                  }
                  frame False {
                  }
                }
              }
            }
          }
          frame "UI: Update CSM Candidates" {
            n136 = call "Read CSMs.vi"() -> ("Array"=w380:string[])  [unwired: 10 in, 1 out]
            n137 = property on="Target" class="CmbBox"("Strings[]"=w380) -> ()  [unwired: 2 in, 2 out]
          }
          frame "UI: Update CSM-VI Candidates" {
            n138 = call "Read CSM-VIs.vi"() -> ("Array"=w385:string[])  [unwired: 10 in, 1 out]
            n139 = property on="CSM-VI" class="CmbBox"("Strings[]"=w385) -> ()  [unwired: 2 in, 2 out]
          }
          frame "UI: Update States Candidates By CSM" {
            n140 = case shown="\"\"" w397 {
              selector: w397 -> [w401 _]
              tunnel: [w401 w402] -> w394
              frame Default {
              }
              frame "" {
                n141 = local read "Target"() -> (w402:string)
              }
            }
            n142 = call "Read CSM Module Info.vi"("CSM Name"=w394) -> ("Cluster"=w391:cluster{"VIName":string})  [unwired: 9 in, 1 out]
            n143 = Unbundle By Name(w391) -> ("VIName"=w390:string)
            n144 = call <vilib>:"Build State String with Arguments__JKI_lib_State_Machine.vi"("Arguments (\"\")"=w390, "State"="UI: Update States Candidates By CSM-VI") -> ("State with Arguments"=w392:string)  [unwired: 4 in]
            n145 = call <vilib>:"Add State(s) to Queue__JKI_lib_State_Machine.vi"("State(s) in Front (\"\")"=w392, "State(s) in (\"\")"=w395) -> ("States Out"=w396:string)  [unwired: 13 in]
          }
          frame "UI: Update States Candidates By CSM-VI" {
            n146 = case shown="\"\"" w410 {
              selector: w410 -> [w415 _]
              tunnel: [w415 w416] -> w409
              frame Default {
              }
              frame "" {
                n147 = local read "CSM-VI"() -> (w416:string)
              }
            }
            n148 = call "Read CSM States By CSM-VI.vi"("CSM VI"=w409) -> ("Array"=w408:string[])  [unwired: 9 in, 1 out]
            n149 = Select(t=enum16{"API-Only", "UserDef States", "All"}."UserDef States" ("Interface-Filter"), s="UserDef State Only", f=enum16{"API-Only", "UserDef States", "All"}."All" ("Interface-Filter")) -> (s? t:f=w403:enum16{"API-Only", "UserDef States", "All"})
            n150 = call "filter CSM States.vi"("Interface-Filter"=w403, "Array"=w408) -> ("filtered array"=w407:string[])  [unwired: 9 in]
            n151 = property on="State" class="CmbBox"("Strings[]"=w407) -> ()  [unwired: 2 in, 2 out]
          }
          frame "UI: Change CSM-VI" {
            n152 = call "Read CSM Module Info.vi"("CSM Name"=w419) -> ("Cluster"=w418:cluster{"VIName":string})  [unwired: 9 in, 1 out]
            n153 = Unbundle By Name(w418) -> ("VIName"=w417:string)
            n154 = local write "CSM-VI"(w417) -> ()
          }
          frame "UI: Change Symbol" {
            n155 = call "Read CSM Module Info.vi"("CSM Name"=w426) -> ("Cluster"=w425:cluster{"VIName":string})  [unwired: 9 in, 1 out]
            n156 = Unbundle By Name(w425) -> ("VIName"=w424:string)
            n157 = local write "CSM-VI"(w424) -> ()
          }
          frame "UI: Update Ctrls State" {
            n158 = local read "Target"() -> (w442:string)
            n159 = control-ref of="State"() -> (w433:refnum<vi>)
            n160 = control-ref of="Argument"() -> (w434:refnum<vi>)
            n161 = control-ref of="symbol"() -> (w435:refnum<vi>)
            n162 = control-ref of="Target"() -> (w436:refnum<vi>)
            n163 = control-ref of="CSM-VI"() -> (w437:refnum<vi>)
            n164 = control-ref of="Comments"() -> (w438:refnum<vi>)
            n165 = To Lower Case(string=w442) -> (all lower case string=w440:string)
            n166 = Search 1D Array(1D array=string[] ["<register>", "<unregister>"], element=w440) -> (index of element=w432:i32)  [unwired: 1 in]
            n167 = Build Array(w433, w434, w435, w436, w437, w438) -> (w439:refnum<vi>[])
            n168 = Greater Or Equal To 0?(x=w432) -> (x >= 0?=w431:bool)
            n169 = for {
              tunnel: w439 -> [w451] mode=indexing
              tunnel: w431 -> [w447]
              n170 = Select(t=T3."Disabled and Grayed Out" ("Disabled"), s=w447, f=T3."Enabled" ("Disabled")) -> (s? t:f=w450:T3)
              n171 = property class="Str"(reference=w451, "DisabledEnum"=w450) -> ()  [unwired: 1 in, 2 out]
            }
          }
          frame "---------- Macro ----------" {
            # "#CSM \"Category Seperator\"\nDo not put any code in this frame."
            n172 = call <vilib>:"Add State(s) to Queue__JKI_lib_State_Machine.vi"("State(s) in (\"\")"=w456) -> ("States Out"=w455:string)  [unwired: 14 in]
          }
          frame "Macro: Initialize" {
            # "#CSM \"Macro: Initialize\"\nInitialization Macro (This is called once, when the VI starts)"
            n173 = call <vilib>:"Add State(s) to Queue__JKI_lib_State_Machine.vi"("State(s) in Front (\"\")"="Data: Initialize\nInitialize Core Data\nEvents: Register\nUI: Initialize\n//UI: Front Panel State >> Open\nUI: Refresh Inputs\nUI: Update CSM Candidates\nUI: Update CSM-VI Candidates\nUI: Update States Candidates By CSM\nUI: Update Ctrls State", "State(s) in (\"\")"=w462) -> ("States Out"=w461:string)  [unwired: 13 in]
          }
          frame "Macro: Exit" {
            # "#CSM \"Macro: Exit\"\nExit Macro (This is called once, when the VI exits)"
            n174 = Unbundle By Name(w471) -> ("Core.Close Panel on Exit?"=w470:bool)
            n175 = Select(t="UI: Front Panel State >> Close", s=w470, f="") -> (s? t:f=w467:string)
            n176 = call <vilib>:"Add State(s) to Queue__JKI_lib_State_Machine.vi"("State(s) in Front (\"\")"="//Exit Sub-Modules ", "State(s) in (\"\")"=w467, "State(s) at Back (\"\")"="Data: Cleanup\nEvents: Unregister\nExit") -> ("States Out"=w465:string)  [unwired: 12 in]
            n177 = call <vilib>:"Add State(s) to Queue__JKI_lib_State_Machine.vi"("State(s) in Front (\"\")"=w465, "State(s) in (\"\")"=w474) -> ("States Out"=w473:string)  [unwired: 13 in]
          }
          frame "---------- API ----------" {
            # "#CSM \"Category Seperator\"\nDo not put any code in this frame."
          }
          frame "API: Set Command" {
            # "#CSM API Example\nCopy/Rename this case for your own API"
            n178 = call "CSM - Revert Arguments-Safe String.vi"("Safe Argument String"=w482) -> ("Origin Argument String"=w483:string)  [unwired: 8 in]
            n179 = Bundle By Name(cluster=w486, "Command"=w483) -> (w484:T8)
            n180 = call <vilib>:"Add State(s) to Queue__JKI_lib_State_Machine.vi"("State(s) in (\"\")"=w480, "State(s) at Back (\"\")"="UI: Refresh Inputs\nUI: Update Ctrls State" ("State(s) in Front (\"\")")) -> ("States Out"=w481:string)  [unwired: 13 in]
          }
          frame "API: Get Command" {
            # "#CSM API Example\nCopy/Rename this case for your own API"
            n181 = local read "State"() -> (w493:string)
            n182 = local read "symbol"() -> (w488:string)
            n183 = local read "Comments"() -> (w497:string)
            n184 = local read "Argument"() -> (w494:string)
            n185 = local read "Target"() -> (w491:string)
            n186 = Concatenate Strings(w493, w488, w491) -> (w492:string)
            n187 = call-poly "Build Message with Arguments++.vi"("State With Arguments"=w492, "Arguments (\"\")"=w494, "Target Module (\"\")"=w491) -> ("CSM Message String"=w498:string)  [unwired: 12 in]
            n188 = case shown="Default" w497 {
              selector: w497 -> [_ w506]
              tunnel: w498 -> [w503 w507]
              tunnel: "  //" ("string") -> [_ w505]
              tunnel: [w503 w504] -> w489
              frame "" {
              }
              frame Default {
                n189 = Concatenate Strings(w507, w505, w506) -> (w504:string)
              }
            }
            n190 = Bundle By Name(cluster=w500, "Command"=w489) -> (w490:T8)
            n191 = call "CSM - Make String Arguments Safe.vi"("Argument String"=w489) -> ("Safe Argument String"=w495:string)  [unwired: 8 in]
          }
          frame "API: Change Symbol" {
            n192 = call "CSM - Revert Arguments-Safe String.vi"("Safe Argument String"=w514) -> ("Origin Argument String"=w508:string)  [unwired: 8 in]
            n193 = local write "symbol"(w508) -> ()
            n194 = Empty String/Path?(string/path=w508) -> (empty?=w510:bool)
            n195 = case shown="True" w510 {
              tunnel: [T3."Enabled" ("Disabled") T3."Disabled and Grayed Out" ("Disabled")] -> w509
              frame False {
              }
              frame True {
              }
            }
            n196 = call-poly "Add State(s) to Queue By BOOL++.vi"("TRUE (\"\")"="API: Change Target >> " ("State(s) in Front (\"\")"), "Condition"=w510, "State Queue (\"\")"=w513) -> ("Remaining States"=w512:string)  [unwired: 8 in]
            n197 = property on="CSM-VI" class="CmbBox"("DisabledEnum"=w509) -> ()  [unwired: 2 in, 2 out]
            n198 = property on="Target" class="CmbBox"("DisabledEnum"=w509) -> ()  [unwired: 2 in, 2 out]
          }
          frame "API: Change Target" {
            n199 = local write "Target"(w520) -> ()
            n200 = call-poly "Build Message with Arguments++.vi"("States With Replace Token"="API: Get Command\nUI: Update States Candidates By CSM >><param>\nUI: Change CSM-VI >><param>\nUI: Update Ctrls State" ("State(s) in Front (\"\")"), "<param>"=w520) -> ("States"=w521:string)  [unwired: 13 in]
            n201 = call <vilib>:"Add State(s) to Queue__JKI_lib_State_Machine.vi"("State(s) in Front (\"\")"=w521, "State(s) in (\"\")"=w523) -> ("States Out"=w527:string)  [unwired: 13 in]
          }
          frame "---------- Action ----------" {
            # "#CSM \"Category Seperator\"\nDo not put any code in this frame."
            n202 = call <vilib>:"Add State(s) to Queue__JKI_lib_State_Machine.vi"("State(s) in (\"\")"=w532) -> ("States Out"=w531:string)  [unwired: 14 in]
          }
        }
      }
      n203 = Unbundle By Name(w10) -> ("Command"=w9:string)
    }
    frame Error {
    }
  }
  "Error Out" <- w4
  "Command Out" <- w1
